vi "Rate scan 8 BITS.vi"(6 "T Ventana":u32 format="%x", 7 "Espera acceso USB":u32, 8 "error in 2":errorcluster, 9 "Valor buscado scalers (5000)":u16, 10 "Sumador":u8, 11 "ftHandle_in 2":u32) -> (0 "error out 2":errorcluster, 1 "Scaler 3\nTH3,TH4,TH5":u16, 2 "Scaler 2\nTH0,TH1,TH2":u16, 3 "ftHandle_out 2":u32, 5 "Scaler 1":u16)   [LabVIEW 2009]
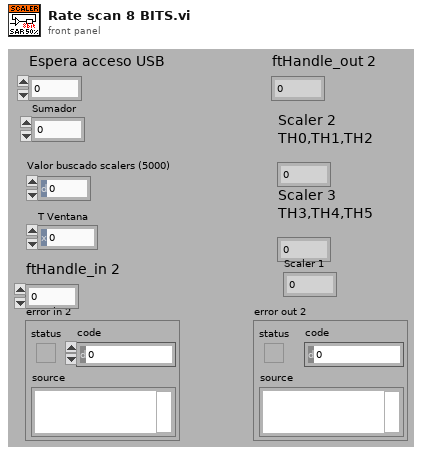
[diagram p1: front panel]
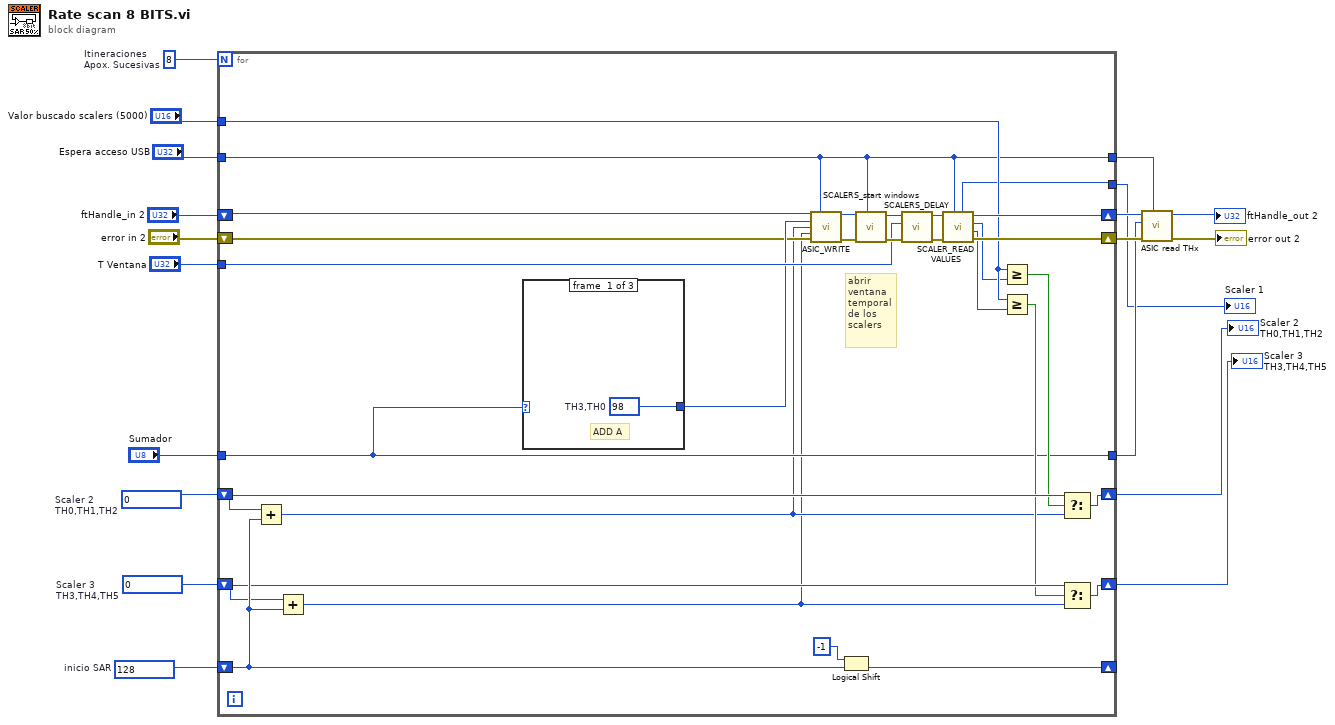
[diagram p0: block diagram]
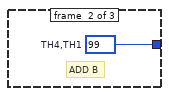
[diagram p2: hidden frame]
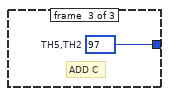
[diagram p3: hidden frame]
diagram:
  w11 = u8 0  # Scaler 3 TH3,TH4,TH5
  w12 = u8 0  # Scaler 2 TH0,TH1,TH2
  w13 = u8 128  # inicio SAR
  w15 = 8  # Itineraciones Apox. Sucesivas
  n1 = for {
    N: w15 -> [_]
    tunnel: "Espera acceso USB" -> [w26]
    tunnel: "T Ventana" -> [w46]
    tunnel: "Valor buscado scalers (5000)" -> [w28]
    shift-right: [w42] -> _
    shift-left: w13 -> [w41]
    shift-right: [w33] -> w2
    shift-left: w12 -> [w38]
    shift-right: [w32] -> w1
    shift-left: w11 -> [w37]
    tunnel: "Sumador" -> [w30]
    shift-right: [w35] -> w8
    shift-left: "ftHandle_in 2" -> [w24]
    shift-right: [w34] -> w9
    shift-left: "error in 2" -> [w23]
    tunnel: [w30] -> w6
    tunnel: [w26] -> w7
    tunnel: [w25] -> w3
    # "abrir ventana temporal de los scalers"
    n2 = Add(x=w38, y=w41) -> (x+y=w22:u8)
    n3 = Add(x=w37, y=w41) -> (x+y=w21:u8)
    n4 = case shown="0, Default" w30 {
      tunnel: [w49 w50 w51] -> w40
      frame #0 {
        w49 = u8 98  # TH3,TH0
        # "ADD A"
      }
      frame #1 {
        w50 = u8 99  # TH4,TH1
        # "ADD B"
      }
      frame #2 {
        w51 = u8 97  # TH5,TH2
        # "ADD C"
      }
    }
    n5 = call "ASIC_WRITE.vi"("ftHandle_in"=w24, "Espera acceso USB"=w26, "Direccion Registro Asic"=w40, "Byte Alto"=w22, "Byte Bajo"=w21, "error in"=w23) -> ("ftHandle_out"=w20:u32, "error out"=w39:errorcluster)  [unwired: 8 in]
    n6 = Logical Shift(y=i8 -1, x=w41) -> (x << y=w42:u8)
    n7 = call "SCALERS_start windows.vi"("Espera acceso USB"=w26, "error in 2"=w39, "ftHandle_in 2"=w20) -> ("error out"=w47:errorcluster, "ftHandle_out"=w48:u32)  [unwired: 7 in]
    n8 = call "SCALERS_DELAY.vi"("error out 2"=w47, "Ventana 2"=w46, "ftHandle_out 2"=w48) -> ("error out"=w44:errorcluster, "ftHandle_out"=w45:u32)  [unwired: 7 in]
    n9 = call "SCALER_READ VALUES.vi"("Espera acceso USB"=w26, "error in"=w44, "ftHandle_in"=w45) -> ("error out"=w34:errorcluster, "Scaler 3"=w29:u16, "Scaler 2"=w27:u16, "ftHandle_out"=w35:u32, "Scaler 1"=w25:u16)  [unwired: 3 in, 1 out]
    n10 = Greater Or Equal?(x=w28, y=w27) -> (x >= y?=w36:bool)
    n11 = Greater Or Equal?(x=w28, y=w29) -> (x >= y?=w31:bool)
    n12 = Select(t=w38, s=w36, f=w22) -> (s? t:f=w33:u8)
    n13 = Select(t=w37, s=w31, f=w21) -> (s? t:f=w32:u8)
  }
  "Scaler 2\nTH0,TH1,TH2" <- w2
  "Scaler 3\nTH3,TH4,TH5" <- w1
  "Scaler 1" <- w3
  n14 = call "ASIC read THx.vi"("Espera acceso USB"=w7, "error in"=w9, "Sumador"=w6, "ftHandle_in"=w8) -> ("error out 2"=→"error out 2":errorcluster, "ftHandle_out 2"=→"ftHandle_out 2":u32)  [unwired: 4 in, 2 out]
